vi "setFolderPermissions.vi"(8 "error in (no error)":errorcluster, 10 "folderPath":path, 11 "FileTransfer in":refnum<class "FileTransfer.lvclass">) -> (0 "error out":errorcluster, 3 "FileTransfer out":refnum<class "FileTransfer.lvclass">)   [LabVIEW 2016, in "FileTransfer.lvclass"]
uses:
  FileTransfer.lvclass
panel:
  out "concatenated string":string
  out "return code":i32
  out "standard error":string
  out "standard output":string
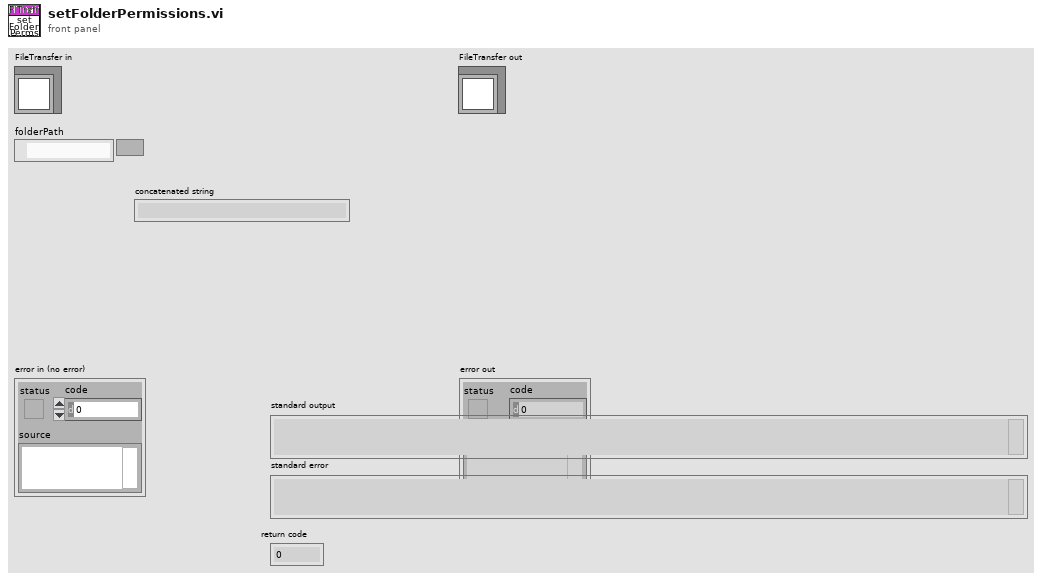
[diagram p1: front panel]
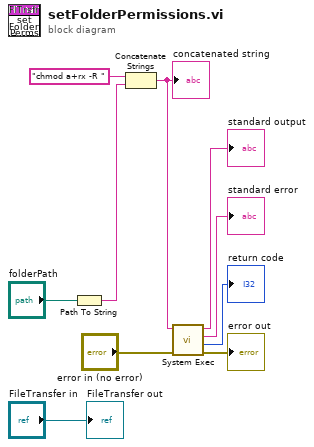
[diagram p0: block diagram]
diagram:
  n1 = Path To String(path="folderPath") -> (string=w5:string)
  n2 = Concatenate Strings("chmod a+rx -R " ("command line"), w5) -> (w10:string)
  "concatenated string" <- w10
  n3 = call <vilib>:"System Exec.vi"("error in (no error)"="error in (no error)", "command line"=w10) -> ("error out"=→"error out":errorcluster, "return code"=→"return code":i32, "standard error"=→"standard error":string, "standard output"=→"standard output":string)  [unwired: 6 in]
  "FileTransfer out" <- "FileTransfer in"
